vi "Main.vi"() -> ()   [LabVIEW 2019]
doc: "This template is for the Queued Message Handler design pattern.\n\nThe Event Handling Loop generates messages based on user interface actions.\n\nThe Message Handling Loop processes messages generated by the Event Handling Loop, or by other messages. The messages are string values, so new messages can be added easily to the Message Cases case structure in the Message Handling Loop. Each message cluster can also provide an optional value for Message Data, which is a variant that can be converted to whatever message-specific data is required."
uses:
  support/Message Queue/Message Cluster.ctl
  controls/UI Refs.ctl
  Settings/Settings.ctl
  Settings/Runtime Conf.ctl
  controls/UI State.ctl
  Acquisition/HeatFlow/HeatFlow Acq Data.ctl
  <extravilib>/ChannelInstances/Stream-var/Read With Abort.vi
  <extravilib>/ChannelInstances/Messenger-t'Message Queue.lvlib-Message Cluster.ctl'/Write With Abort.vi
  <extravilib>/ChannelInstances/Stream-var/EndpointRead.vi
  <resource>/Channels/Messenger/Write With Abort.vi
  <extravilib>/ChannelInstances/Messenger-t'Message Queue.lvlib-Message Cluster.ctl'/Wrapper.lvclass
  C:/Program Files (x86)/National Instruments/LabVIEW 2019/vi.lib/ChannelSupport/Channel Message/Channel Message.lvclass
  <extravilib>/ChannelInstances/Stream-var/Instantiate.vi
  <extravilib>/ChannelInstances/Stream-var/)Channel.vi
  <resource>/ChannelSupport/_ChannelSupport/WaitIfNeeded.vi
  <extravilib>/ChannelInstances/Messenger-t'Message Queue.lvlib-Message Cluster.ctl'/Instantiate.vi
  <extravilib>/ChannelInstances/Messenger-t'Message Queue.lvlib-Message Cluster.ctl'/Wrap.vi
  <resource>/Channels/Messenger/Endpoint.vi
  <extravilib>/ChannelInstances/Event Messenger-bool/Instantiate.vi
  <extravilib>/ChannelInstances/Event Messenger-bool/))Channel.vi
  <vilib>/Utility/error.llb/Error Cluster From Error Code.vi
  <vilib>/ErrorRing/Error Ring.xnode
  <extravilib>/ChannelInstances/Event Messenger-bool.lvlib
  support/Message Queue/Message Queue.lvlib
  <extravilib>/ChannelInstances/Messenger-t'Message Queue.lvlib-Message Cluster.ctl'.lvlib
  Settings/Settings.lvlib
  Acquisition/Acquisition.lvlib
  Logging/Logging.lvlib
  <extravilib>/ChannelInstances/Stream-var.lvlib
panel:
  out "Jaka wartoœæ":dbl
  in  "ColdSideVolts":dbl min=0.0 max=8.0 step=0.01
  in  "HotSideVolts":dbl min=0.0 max=8.0 step=0.01
  out "Operating Mode":string
  in  "Tab Control":enum32{"Page 1", "Page 2"}(tab)
  out "Heater dU":dbl format="%#.3f"
  out "Hot Side I":dbl format="%#.3f"
  out "I Res dU":dbl format="%#.1f"
  in  "Load Resistance":dbl=3.0 min=0.01 max=100000.0 step=1.0 format="%#.2f"
  out "Load Voltage":dbl format="%#.2f"
  in  "R Check":dbl=5.0 min=0.01 max=100000.0 step=1.0 format="%#.2f"
  in  "s":bool
  out "Boolean":bool
  out "Boolean 2":bool
  in  "s 2":bool
  out "Boolean 3":bool
  out "Boolean 4":bool
  out "Output Power":dbl format="%#.2f"
  out "Output Current":dbl format="%#.0f"
  out "Current above limit":bool
  out "Hot Side Power":dbl format="%9.2f"
  out "Hot Side Temp":dbl format="%#.2f"
  out "Cold Side Temp":dbl format="%#.2f"
  out "T 1":dbl
  out "T 2":dbl
  out "T 3":dbl
  out "T 4":dbl
  out "T 5":dbl
  out "T 6":dbl
  out "T 7":dbl
  out "T 8":dbl
  out "Time Stamp":timestamp
  out "Time Delta ms":u32
  in  "Save Conf File":bool
  out "Config File":string
  in  "Select Config File":bool
  out "Status":string
  out "Current Time Interval, s":dbl
  in  "Update Runtime":bool
  in  "Time Interval, s":dbl=1.0
  in  "Stop Acquisition":bool
  in  "Log all signals":bool
  in  "Start Acquisition":bool
  in  "Exit":bool
  # "K"
  # "K"
  # "W"
  # "mV"
  # "A"
  # "V"
  # "V"
  # "Ohm"
  # "Pomiar Rw"
  # "10 000 Ohm"
  # "W"
  # "Ohm"
  # "mA"
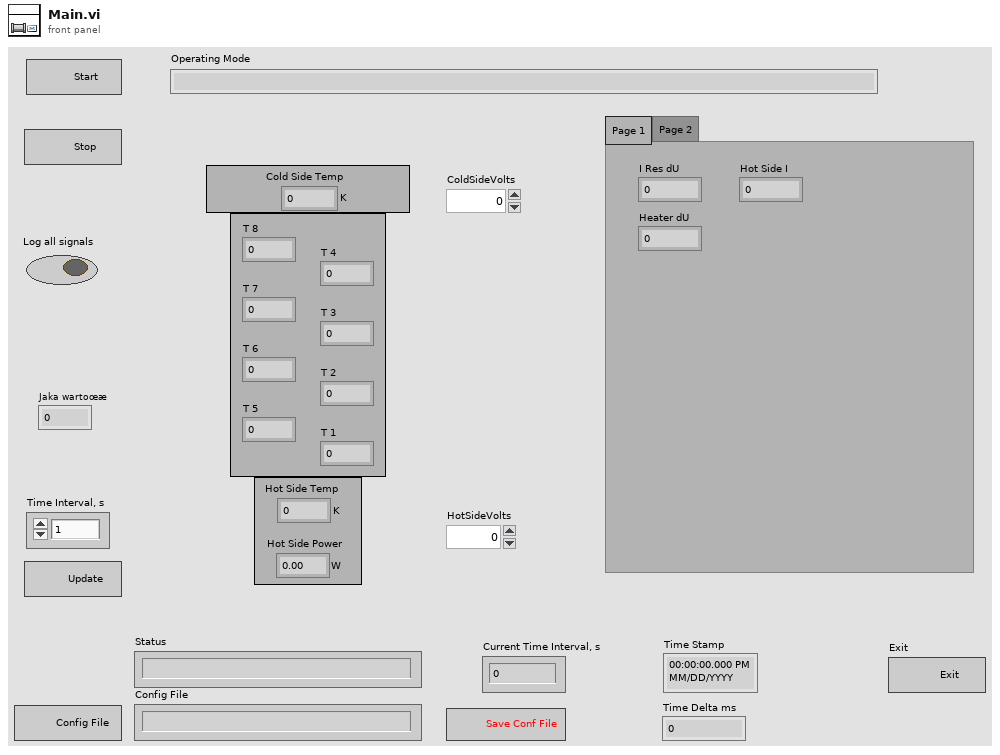
[diagram p1: front panel]
types:
  T1 = typedef "UI State.ctl" = enum16{"Idle", "Acquiring and Logging", "Waiting for Exit", "Waiting for Exit (Acq Stopped)", "Waiting for Exit (Log Stopped)", "Waiting for Stop", "Waiting for Stop (Acq Stopped)", "Waiting for Stop (Log Stopped)"}
  T2 = typedef "Settings.lvlib/Settings.ctl" = cluster{"Runtime":T3, "Cfg Files Dir":path, "Cfg File":path}
  T3 = typedef "Settings.lvlib/Runtime Conf.ctl" = cluster{"Time Interval, s":dbl, "Time Resolution, ms":u32, "Hot Side MOS, V":dbl, "Cold Side MOS, V":dbl}
  T4 = typedef "UI Refs.ctl" = cluster{"Start Acq Ref":refnum<vi>, "Log All Ref":refnum<vi>, "Exit Ref":refnum<vi>, "Stop Acq Ref":refnum<vi>, "Update Ref":refnum<vi>, "Select Config File":refnum<vi>, "Save Config File":refnum<vi>}
  T5 = typedef "Message Queue.lvlib/Message Cluster.ctl" = cluster{"Message":string, "Message Data":variant}
  T6 = typedef "Messenger-t'Message Queue.lvlib-Message Cluster.ctl'.lvlib/))Channel.ctl" = refnum<queue>
  T7 = typedef "Event Messenger-bool.lvlib/))Channel.ctl" = refnum<queue>
  T8 = typedef "Stream-var.lvlib/)Channel.ctl" = refnum<queue>
  T9 = typedef "Acquisition.lvlib/HeatFlow Acq Data.ctl" = cluster{"Time Stamp":timestamp, "Time Delta":u32, "LakeShore_Temp":cluster{"Tube_T_1":dbl, "Tube_T_2":dbl, "Tube_T_3":dbl, "Tube_T_4":dbl, "Tube_T_5":dbl, "Tube_T_6":dbl, "Tube_T_7":dbl, "Tube_T_8":dbl}, "Heaters":cluster{"I_Res_dU":dbl, "Heater_dU":dbl, "Hot_Side_I":dbl, "Hot_Side_P":dbl, "Cold_Ctrl_U":dbl, "Hot_Ctrl_U":dbl, "Hot_Side_T":dbl, "Cold_Side_T":dbl}, "TEG":cluster{"TEG_Load_dU":dbl, "TEG_Load_R":dbl, "TEG_Load_I":dbl, "TEG_Load_P":dbl, "TEG_eta":dbl, "TEG_dT":dbl, "TEG_U_open":dbl, "TEG_U_Test":dbl, "TEG_R_Test":dbl, "TEG_Rw":dbl}, "LastElement?":bool}
  T10 = cluster{"Tube_T_1":dbl, "Tube_T_2":dbl, "Tube_T_3":dbl, "Tube_T_4":dbl, "Tube_T_5":dbl, "Tube_T_6":dbl, "Tube_T_7":dbl, "Tube_T_8":dbl}
  T11 = cluster{"I_Res_dU":dbl, "Heater_dU":dbl, "Hot_Side_I":dbl, "Hot_Side_P":dbl, "Cold_Ctrl_U":dbl, "Hot_Ctrl_U":dbl, "Hot_Side_T":dbl, "Cold_Side_T":dbl}
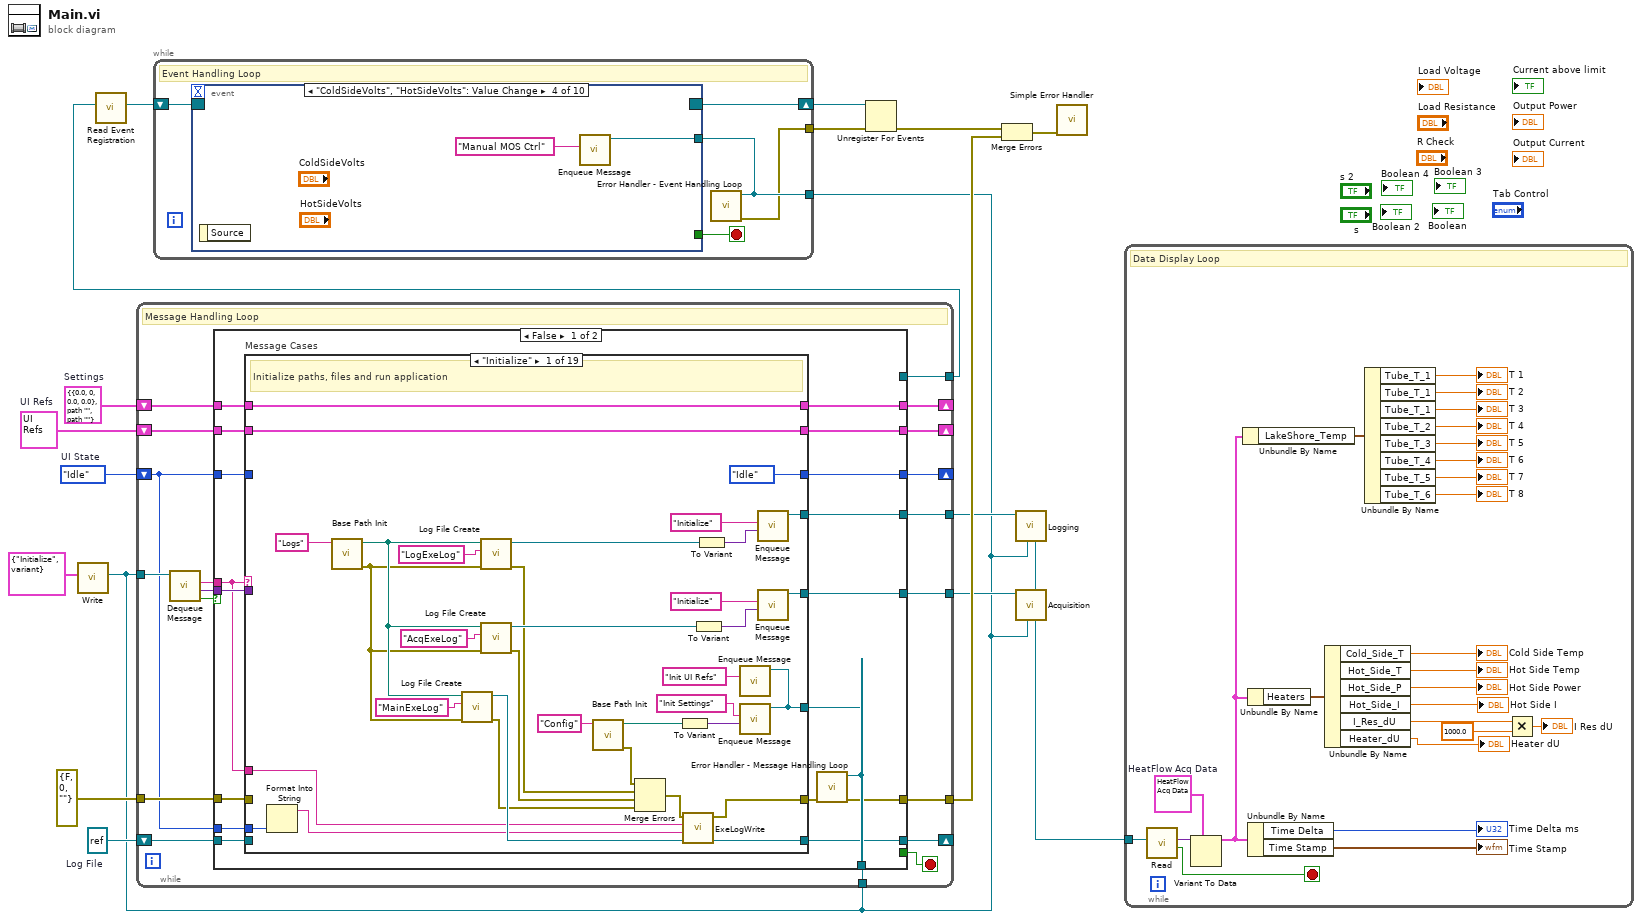
[diagram p0: block diagram]
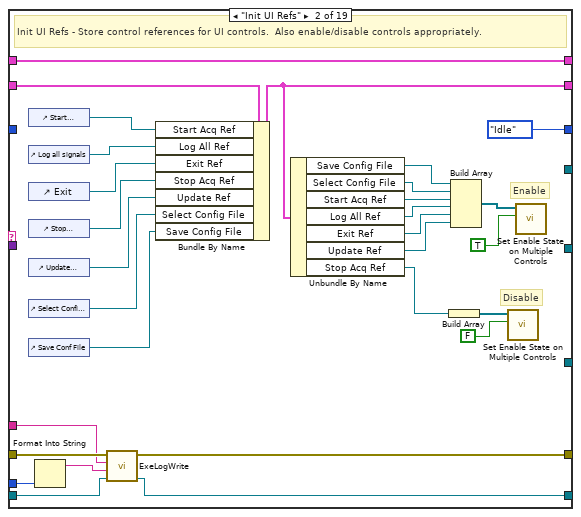
[diagram p2: hidden frame]
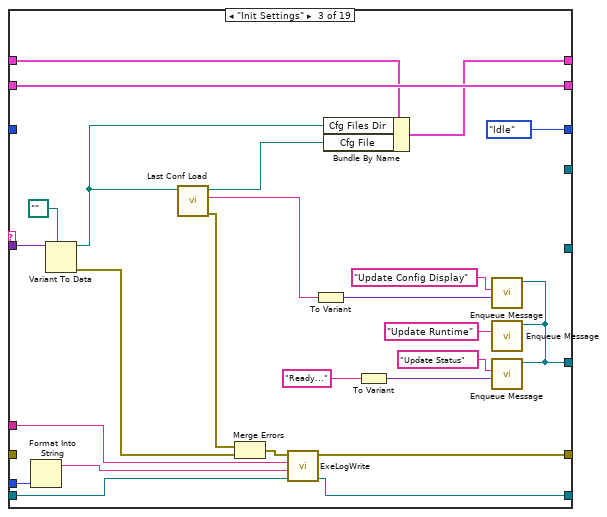
[diagram p3: hidden frame]
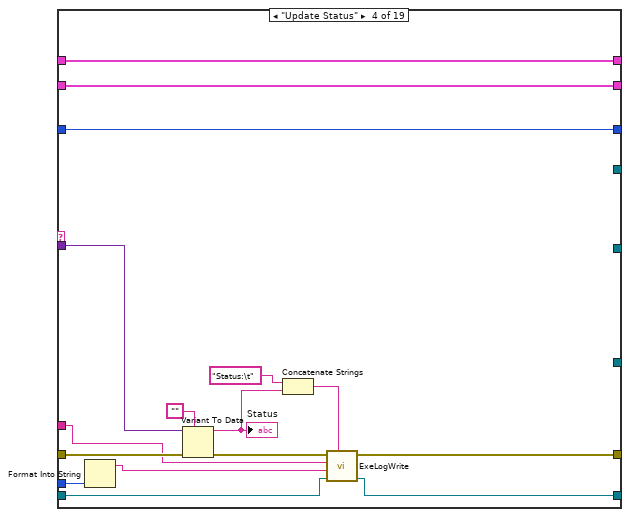
[diagram p4: hidden frame]
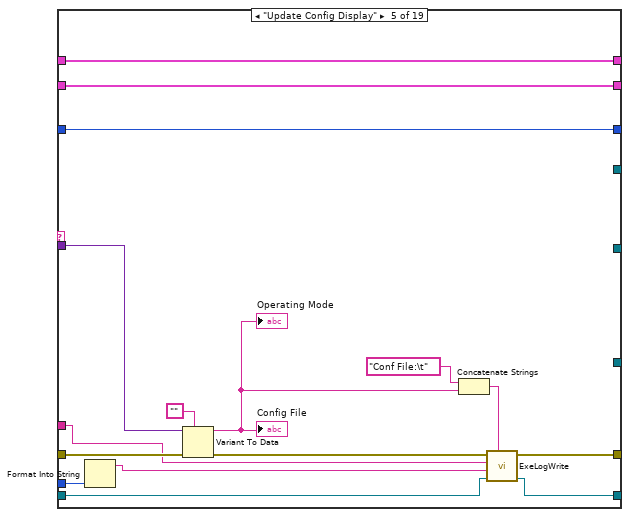
[diagram p5: hidden frame]
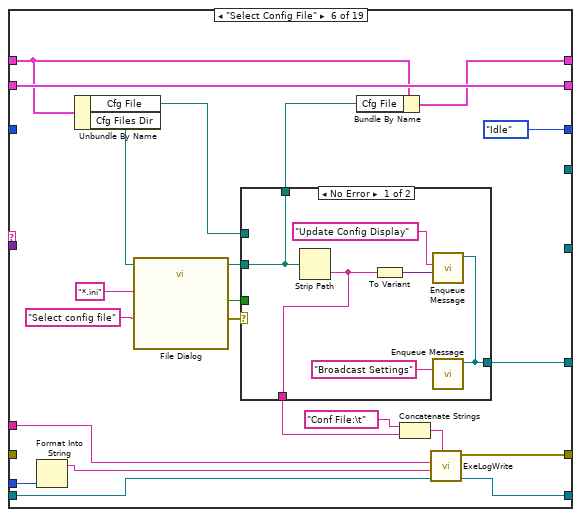
[diagram p6: hidden frame]
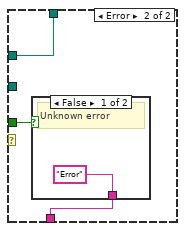
[diagram p7: hidden frame]
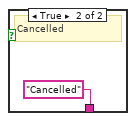
[diagram p8: hidden frame]
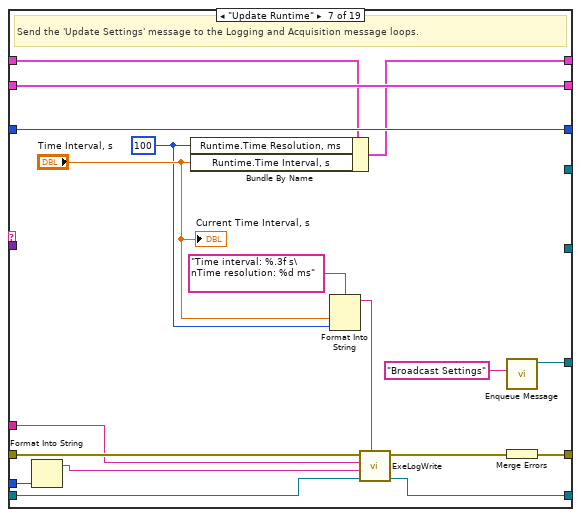
[diagram p9: hidden frame]
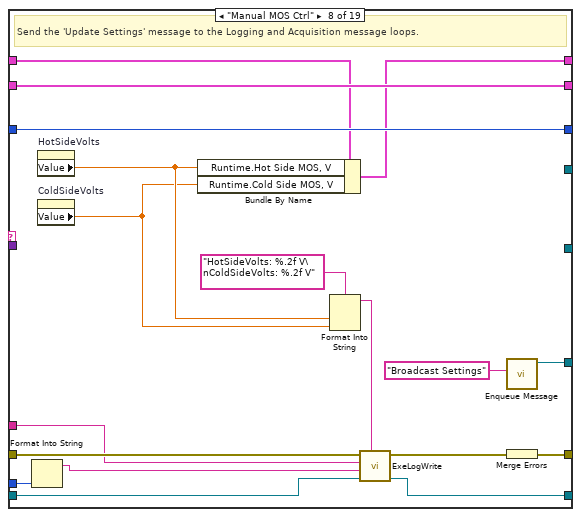
[diagram p10: hidden frame]
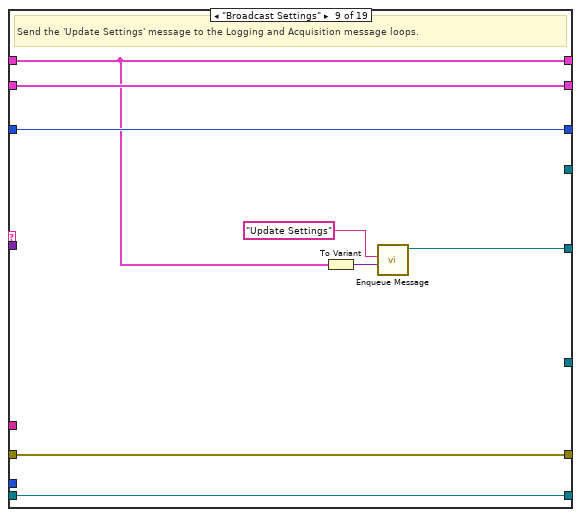
[diagram p11: hidden frame]
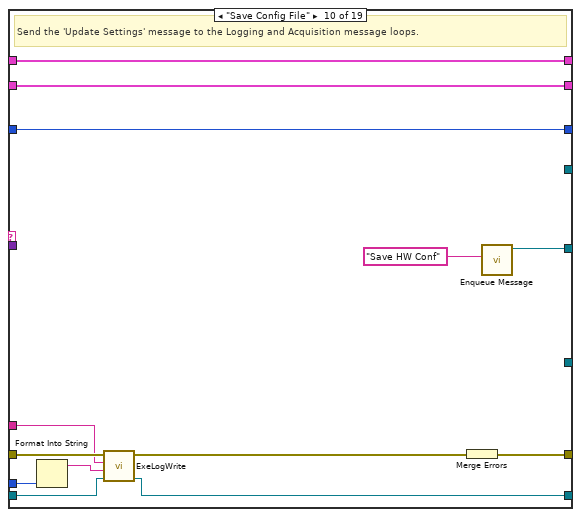
[diagram p12: hidden frame]
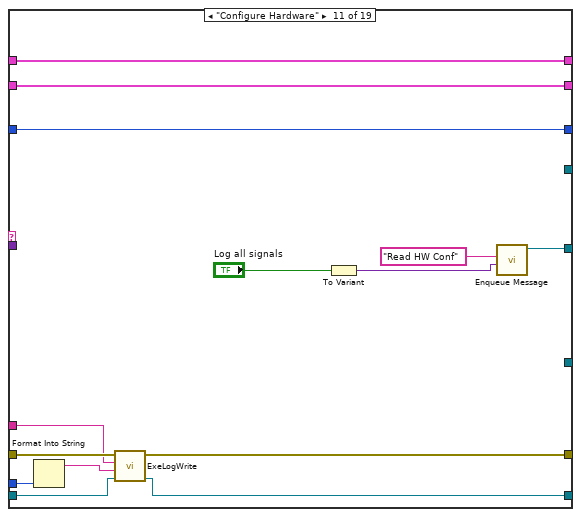
[diagram p13: hidden frame]
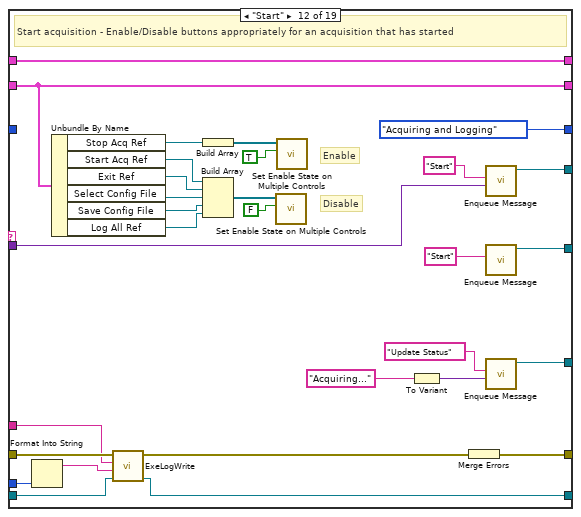
[diagram p14: hidden frame]
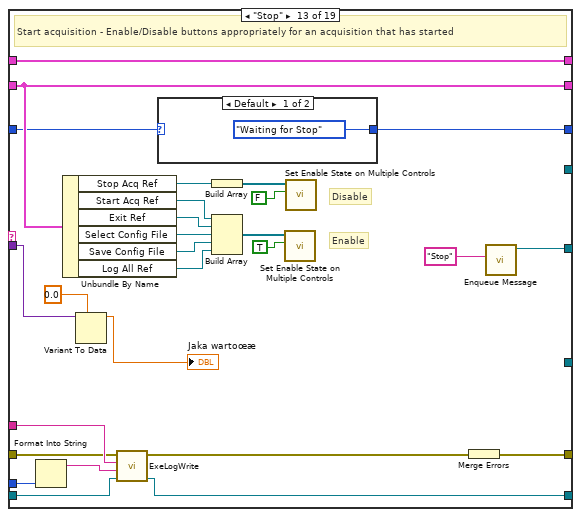
[diagram p15: hidden frame]
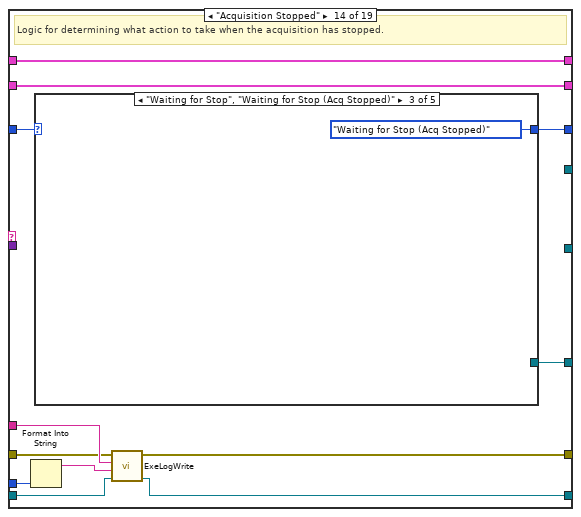
[diagram p17: hidden frame]
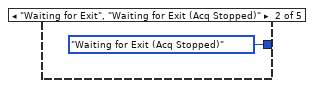
[diagram p19: hidden frame]
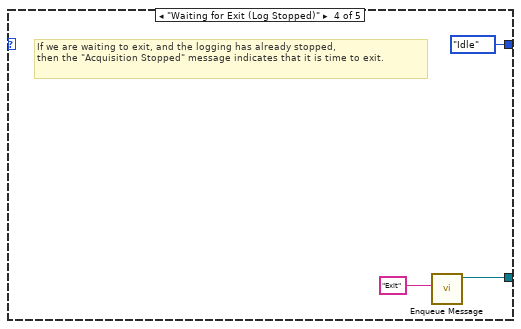
[diagram p20: hidden frame]
diagram:
  w5 = refnum<file> refnum  # Log File
  w10 = UI_State."Idle"  # UI State
  w11 = T2 {"Runtime"={"Time Interval, s"=0.0, "Time Resolution, ms"=0, "Hot Side MOS, V"=0.0, "Cold Side MOS, V"=0.0}, "Cfg Files Dir"=path "", "Cfg File"=path ""}  # Settings
  w12 = T4 {"Start Acq Ref"=refnum, "Log All Ref"=refnum, "Exit Ref"=refnum, "Stop Acq Ref"=refnum, "Update Ref"=refnum, "Select Config File"=refnum, "Save Config File"=refnum}  # UI Refs
  n1 = call <extravilib>:"Write.vi"("element"=T5 {"Message"="Initialize", "Message Data"=variant}) -> ("channel"=w3:T6)  [unwired: 8 in, 2 out]
  n2 = while {
    tunnel: [w37] -> w9
    tunnel: [w36] -> w16
    tunnel: w3 -> [w33]
    tunnel: errorcluster {"status"=FALSE, "code"=0, "source"=""} ("error IO") -> [w35]
    tunnel: w3 -> [w34]
    shift-right: [w28] -> _
    shift-left: w12 -> [w29]
    shift-right: [w26] -> _
    shift-left: w11 -> [w27]
    shift-right: [w25] -> _
    shift-left: w10 -> [w21]
    tunnel: [w24] -> w4
    tunnel: [w23] -> w7
    shift-right: [w19] -> _
    shift-left: w5 -> [w20]
    stop <- w22 stop-if-true
    # "Message Handling Loop"
    n3 = call "Dequeue Message.vi"("channel"=w33) -> ("channel aborted"=w30:bool, "message data"=w31:variant, "message"=w32:string)  [unwired: 8 in]
    n4 = case shown="False" w30 {
      tunnel: [_ TRUE] -> w22
      tunnel: [w54 w471] -> w37
      tunnel: [_ w478] -> w36
      tunnel: w32 -> [w41 _]
      tunnel: w31 -> [w52 w480]
      tunnel: w35 -> [w51 w472]
      tunnel: [w50 _] -> w34
      tunnel: w29 -> [w49 w477]
      tunnel: [w48 w477] -> w28
      tunnel: w27 -> [w47 w476]
      tunnel: [w46 w476] -> w26
      tunnel: w21 -> [w45 w475]
      tunnel: [w44 w475] -> w25
      tunnel: [w43 _] -> w24
      tunnel: [w42 _] -> w23
      tunnel: w21 -> [w38 w474]
      tunnel: w20 -> [w40 w470]
      tunnel: [w39 w469] -> w19
      frame False {
        n5 = case "Message Cases" shown="\"Initialize\"" w41 {
          selector: w41 -> [_ _ _ _ _ _ _ _ _ _ _ _ _ _ _ _ _ _ w459]
          tunnel: w51 -> [_ w98 _ w156 w172 _ w218 w236 w245 w258 w275 w289 w319 w341 w363 _ w405 _ _]
          tunnel: [w59 w93 w127 w150 w166 w189 w225 w243 w245 w264 w274 w308 w335 w339 w361 w396 w404 w440 w460] -> w53
          tunnel: w52 -> [_ _ w138 w157 w173 _ _ _ _ _ _ w281 w311 _ _ w398 _ _ _]
          tunnel: [w84 _ w118 _ _ w179 w208 w228 _ _ _ w294 _ w345 w367 w382 w409 w444 _] -> w50
          tunnel: w49 -> [w87 w115 w140 w155 w171 w196 w224 w242 w251 w263 w268 w302 w331 w348 w370 w395 w412 w445 w458]
          tunnel: [w87 w108 w140 w155 w171 w196 w224 w242 w251 w263 w268 w302 w331 w348 w370 w395 w412 w445 w458] -> w48
          tunnel: w47 -> [w58 w117 w125 w154 w170 w186 w221 w239 w246 w252 w269 w306 w333 w349 w371 w394 w413 w435 w457]
          tunnel: [w58 w117 w124 w154 w170 w185 w220 w238 w246 w252 w269 w306 w333 w349 w371 w394 w413 w435 w457] -> w46
          tunnel: w45 -> [_ _ _ w153 w169 _ w223 w241 w250 w262 w267 _ w324 w347 w369 w393 w411 _ w456]
          tunnel: [UI_State."Idle" ("UI State") UI_State."Idle" ("UI State") UI_State."Idle" ("UI State") w153 w169 UI_State."Idle" ("UI State") w223 w241 w250 w262 w267 UI_State."Acquiring and Logging" ("UI State") w323 w346 w368 w393 w410 UI_State."Idle" ("UI State") w456] -> w44
          tunnel: [w82 _ _ _ _ _ _ _ w249 w261 w277 w303 w332 _ _ _ _ w452 _] -> w43
          tunnel: [w83 _ _ _ _ _ _ _ _ _ _ w304 _ _ _ _ _ w453 _] -> w42
          tunnel: w41 -> [w62 w97 w135 w149 w165 w193 w214 w232 _ w257 w273 w287 w320 w342 w364 w390 w406 w441 _]
          tunnel: w40 -> [_ w95 w133 w147 w163 w191 w216 w234 w244 w255 w271 w285 w317 w340 w362 w389 w403 w439 w455]
          tunnel: [w67 w94 w132 w146 w162 w190 w215 w233 w244 w253 w270 w284 w316 w338 w360 w388 w402 w438 w455] -> w39
          tunnel: w38 -> [w64 w99 w137 w152 w168 w194 w219 w237 _ w259 w276 w290 w322 w344 w366 w392 w408 w443 _]
          frame "Initialize" {
            # "Initialize paths, files and run application"
            n6 = Format Into String(w64) -> (resulting string=w63:string)  [unwired: 3 in, 1 out]
            n7 = call "Base Path Init.vi"("Folder name"="Logs" ("name or relative path")) -> ("error out"=w65:errorcluster, "Folder Path"=w69:path)  [unwired: 9 in]
            n8 = call "Log File Create.vi"("error in"=w65, "initial filename"="MainExeLog", "base path"=w69) -> ("error out"=w61:errorcluster, "refnum out"=w66:refnum<file>)  [unwired: 7 in]
            n9 = call "Log File Create.vi"("error in"=w65, "initial filename"="LogExeLog", "base path"=w69) -> ("error out"=w56:errorcluster, "refnum out"=w78:refnum<file>)  [unwired: 7 in]
            n10 = call "Log File Create.vi"("error in"=w65, "initial filename"="AcqExeLog", "base path"=w69) -> ("error out"=w57:errorcluster, "refnum out"=w76:refnum<file>)  [unwired: 7 in]
            n11 = call "Base Path Init.vi"("Folder name"="Config") -> ("error out"=w55:errorcluster, "Folder Path"=w71:path)  [unwired: 9 in]
            n12 = Merge Errors(w55, w56, w57, w61) -> (w60:errorcluster)
            n13 = To Variant(anything=w71) -> (Variant=w70:variant)
            n14 = call "ExeLogWrite.vi"("refnum in"=w66, "State"=w63, "Message"=w62, "error in"=w60) -> ("refnum out"=w67:refnum<file>, "error out"=w59:errorcluster)  [unwired: 6 in]
            n15 = To Variant(anything=w76) -> (Variant=w74:variant)
            n16 = To Variant(anything=w78) -> (Variant=w75:variant)
            n17 = call "Enqueue Message.vi"("data (empty)"=w70, "message"="Init Settings" ("Message")) -> ("channel"=w84:T6)  [unwired: 9 in]
            n18 = call "Enqueue Message.vi"("channel"=w84, "message"="Init UI Refs" ("Message")) -> ()  [unwired: 10 in]
            n19 = call "Enqueue Message.vi"("data (empty)"=w75, "message"="Initialize") -> ("channel"=w83:T6)  [unwired: 9 in]
            n20 = call "Enqueue Message.vi"("data (empty)"=w74, "message"="Initialize") -> ("channel"=w82:T6)  [unwired: 9 in]
          }
          frame "Init UI Refs" {
            # "Enable"
            # "Disable"
            # "Init UI Refs - Store control references for UI controls.  Also enable/disable controls appropriately."
            n21 = control-ref of="Start Acquisition"() -> (w114:refnum<vi>)
            n22 = control-ref of="Log all signals"() -> (w113:refnum<vi>)
            n23 = control-ref of="Exit"() -> (w110:refnum<vi>)
            n24 = control-ref of="Stop Acquisition"() -> (w109:refnum<vi>)
            n25 = control-ref of="Update Runtime"() -> (w92:refnum<vi>)
            n26 = control-ref of="Select Config File"() -> (w91:refnum<vi>)
            n27 = control-ref of="Save Conf File"() -> (w90:refnum<vi>)
            n28 = Format Into String(w99) -> (resulting string=w96:string)  [unwired: 3 in, 1 out]
            n29 = call "ExeLogWrite.vi"("refnum in"=w95, "State"=w96, "Message"=w97, "error in"=w98) -> ("refnum out"=w94:refnum<file>, "error out"=w93:errorcluster)  [unwired: 6 in]
            n30 = Bundle By Name(cluster=w115, "Start Acq Ref"=w114, "Log All Ref"=w113, "Exit Ref"=w110, "Stop Acq Ref"=w109, "Update Ref"=w92, "Select Config File"=w91, "Save Config File"=w90) -> (w108:T4)
            n31 = Unbundle By Name(w108) -> ("Save Config File"=w89:refnum<vi>, "Select Config File"=w100:refnum<vi>, "Start Acq Ref"=w104:refnum<vi>, "Log All Ref"=w103:refnum<vi>, "Exit Ref"=w102:refnum<vi>, "Update Ref"=w101:refnum<vi>, "Stop Acq Ref"=w107:refnum<vi>)
            n32 = Build Array(w107) -> (w106:refnum<vi>[])
            n33 = Build Array(w89, w100, w104, w103, w102, w101) -> (w105:refnum<vi>[])
            n34 = call "Set Enable State on Multiple Controls.vi"("Enable?"=FALSE, "Controls"=w106) -> ()  [unwired: 10 in]
            n35 = call "Set Enable State on Multiple Controls.vi"("Enable?"=TRUE, "Controls"=w105) -> ()  [unwired: 10 in]
          }
          frame "Init Settings" {
            n36 = Format Into String(w137) -> (resulting string=w134:string)  [unwired: 3 in, 1 out]
            n37 = Variant To Data(type=path "" ("Folder Path"), Variant=w138) -> (data=w123:path, error out=w120:errorcluster)  [unwired: 1 in]
            n38 = call "Last Conf Load.vi"("Config Dir"=w123) -> ("error out"=w119:errorcluster, "Conf File Name"=w121:string, "Conf File path"=w122:path)  [unwired: 8 in]
            n39 = Merge Errors(w119, w120) -> (w126:errorcluster)
            n40 = call "ExeLogWrite.vi"("refnum in"=w133, "State"=w134, "Message"=w135, "error in"=w126) -> ("refnum out"=w132:refnum<file>, "error out"=w127:errorcluster)  [unwired: 6 in]
            n41 = To Variant(anything=w121) -> (Variant=w130:variant)
            n42 = Bundle By Name(cluster=w125, "Cfg Files Dir"=w123, "Cfg File"=w122) -> (w124:T2)
            n43 = To Variant(anything="Ready...") -> (Variant=w129:variant)
            n44 = call "Enqueue Message.vi"("data (empty)"=w129, "message"="Update Status" ("Message")) -> ("channel"=w118:T6)  [unwired: 9 in]
            n45 = call "Enqueue Message.vi"("channel"=w118, "data (empty)"=w130, "message"="Update Config Display") -> ()  [unwired: 9 in]
            n46 = call "Enqueue Message.vi"("channel"=w118, "message"="Update Runtime" ("Message")) -> ()  [unwired: 10 in]
          }
          frame "Update Status" {
            n47 = Format Into String(w152) -> (resulting string=w148:string)  [unwired: 3 in, 1 out]
            n48 = Variant To Data(error in=w156, type="", Variant=w157) -> (data=w144:string, error out=w151:errorcluster)
            "Status" <- w144
            n49 = Concatenate Strings("Status:\t" ("string"), w144) -> (w143:string)
            n50 = call "ExeLogWrite.vi"("Extra"=w143, "refnum in"=w147, "State"=w148, "Message"=w149, "error in"=w151) -> ("refnum out"=w146:refnum<file>, "error out"=w150:errorcluster)  [unwired: 5 in]
          }
          frame "Update Config Display" {
            n51 = Format Into String(w168) -> (resulting string=w164:string)  [unwired: 3 in, 1 out]
            n52 = Variant To Data(error in=w172, type="", Variant=w173) -> (data=w159:string, error out=w167:errorcluster)
            "Config File" <- w159
            "Operating Mode" <- w159
            n53 = Concatenate Strings("Conf File:\t" ("string"), w159) -> (w160:string)
            n54 = call "ExeLogWrite.vi"("Extra"=w160, "refnum in"=w163, "State"=w164, "Message"=w165, "error in"=w167) -> ("refnum out"=w162:refnum<file>, "error out"=w166:errorcluster)  [unwired: 5 in]
          }
          frame "Select Config File" {
            n55 = Format Into String(w194) -> (resulting string=w192:string)  [unwired: 3 in, 1 out]
            n56 = Unbundle By Name(w186) -> ("Cfg File"=w181:path, "Cfg Files Dir"=w183:path)
            n57 = call "File Dialog"("start path"=w183, "prompt"="Select config file", "pattern (all files)"="*.ini") -> ("selected path"=w182:path, "cancelled"=w175:bool, "error out"=w184:errorcluster)  [unwired: 9 in, 1 out]
            n58 = case shown="No Error" w184 {
              tunnel: w182 -> [w198 _]
              tunnel: w181 -> [_ w205]
              tunnel: [w198 w205] -> w180
              tunnel: [w199 _] -> w179
              tunnel: [w197 w203] -> w177
              tunnel: w175 -> [_ w204]
              frame No Error {
                n59 = Strip Path(path=w198) -> (name=w197:string)  [unwired: 1 out]
                n60 = To Variant(anything=w197) -> (Variant=w200:variant)
                n61 = call "Enqueue Message.vi"("message"="Broadcast Settings") -> ("channel"=w199:T6)  [unwired: 10 in]
                n62 = call "Enqueue Message.vi"("channel"=w199, "data (empty)"=w200, "message"="Update Config Display") -> ()  [unwired: 9 in]
              }
              frame Error {
                n63 = case shown="False" w204 {
                  tunnel: ["Error" "Cancelled"] -> w203
                  frame False {
                    # "Unknown error"
                  }
                  frame True {
                    # "Cancelled"
                  }
                }
              }
            }
            n64 = Bundle By Name(cluster=w186, "Cfg File"=w180) -> (w185:T2)
            n65 = Concatenate Strings("Conf File:\t" ("string"), w177) -> (w176:string)
            n66 = call "ExeLogWrite.vi"("Extra"=w176, "refnum in"=w191, "State"=w192, "Message"=w193) -> ("refnum out"=w190:refnum<file>, "error out"=w189:errorcluster)  [unwired: 6 in]
          }
          frame "Update Runtime" {
            w211 = u32 100 ("Runtime Configuration.Time Resolution, ms")
            # "Send the 'Update Settings' message to the Logging and Acquisition message loops."
            n67 = Format Into String(w219) -> (resulting string=w213:string)  [unwired: 3 in, 1 out]
            n68 = Bundle By Name(cluster=w221, "Runtime.Time Resolution, ms"=w211, "Runtime.Time Interval, s"="Time Interval, s") -> (w220:T2)
            n69 = Format Into String(format string="Time interval: %.3f s\nTime resolution: %d ms", "Time Interval, s", w211) -> (resulting string=w209:string)  [unwired: 2 in, 1 out]
            n70 = call "ExeLogWrite.vi"("Extra"=w209, "refnum in"=w216, "State"=w213, "Message"=w214, "error in"=w218) -> ("refnum out"=w215:refnum<file>, "error out"=w217:errorcluster)  [unwired: 5 in]
            n71 = call "Enqueue Message.vi"("message"="Broadcast Settings") -> ("channel"=w208:T6)  [unwired: 10 in]
            n72 = Merge Errors(w217) -> (w225:errorcluster)
            "Current Time Interval, s" <- "Time Interval, s"
          }
          frame "Manual MOS Ctrl" {
            # "Send the 'Update Settings' message to the Logging and Acquisition message loops."
            n73 = Format Into String(w237) -> (resulting string=w231:string)  [unwired: 3 in, 1 out]
            n74 = property on="HotSideVolts" class="DigNum (strict)"() -> ("Value"=w227:dbl)  [unwired: 2 in, 2 out]
            n75 = property on="ColdSideVolts" class="DigNum (strict)"() -> ("Value"=w226:dbl)  [unwired: 2 in, 2 out]
            n76 = Bundle By Name(cluster=w239, "Runtime.Hot Side MOS, V"=w227, "Runtime.Cold Side MOS, V"=w226) -> (w238:T2)
            n77 = Format Into String(format string="HotSideVolts: %.2f V\nColdSideVolts: %.2f V", w227, w226) -> (resulting string=w229:string)  [unwired: 2 in, 1 out]
            n78 = call "ExeLogWrite.vi"("Extra"=w229, "refnum in"=w234, "State"=w231, "Message"=w232, "error in"=w236) -> ("refnum out"=w233:refnum<file>, "error out"=w235:errorcluster)  [unwired: 5 in]
            n79 = call "Enqueue Message.vi"("message"="Broadcast Settings") -> ("channel"=w228:T6)  [unwired: 10 in]
            n80 = Merge Errors(w235) -> (w243:errorcluster)
          }
          frame "Broadcast Settings" {
            # "Send the 'Update Settings' message to the Logging and Acquisition message loops."
            n81 = To Variant(anything=w246) -> (Variant=w247:variant)
            n82 = call "Enqueue Message.vi"("data (empty)"=w247, "message"="Update Settings") -> ("channel"=w249:T6)  [unwired: 9 in]
          }
          frame "Save Config File" {
            # "Send the 'Update Settings' message to the Logging and Acquisition message loops."
            n83 = Format Into String(w259) -> (resulting string=w256:string)  [unwired: 3 in, 1 out]
            n84 = call "ExeLogWrite.vi"("refnum in"=w255, "State"=w256, "Message"=w257, "error in"=w258) -> ("refnum out"=w253:refnum<file>, "error out"=w254:errorcluster)  [unwired: 6 in]
            n85 = Merge Errors(w254) -> (w264:errorcluster)
            n86 = call "Enqueue Message.vi"("message"="Save HW Conf") -> ("channel"=w261:T6)  [unwired: 10 in]
          }
          frame "Configure Hardware" {
            n87 = Format Into String(w276) -> (resulting string=w272:string)  [unwired: 3 in, 1 out]
            n88 = call "ExeLogWrite.vi"("refnum in"=w271, "State"=w272, "Message"=w273, "error in"=w275) -> ("refnum out"=w270:refnum<file>, "error out"=w274:errorcluster)  [unwired: 6 in]
            n89 = To Variant(anything="Log all signals") -> (Variant=w265:variant)
            n90 = call "Enqueue Message.vi"("data (empty)"=w265, "message"="Read HW Conf" ("Message")) -> ("channel"=w277:T6)  [unwired: 9 in]
          }
          frame "Start" {
            # "Disable"
            # "Enable"
            # "Start acquisition - Enable/Disable buttons appropriately for an acquisition that has started"
            n91 = Format Into String(w290) -> (resulting string=w286:string)  [unwired: 3 in, 1 out]
            n92 = Unbundle By Name(w302) -> ("Stop Acq Ref"=w301:refnum<vi>, "Start Acq Ref"=w298:refnum<vi>, "Exit Ref"=w283:refnum<vi>, "Select Config File"=w282:refnum<vi>, "Save Config File"=w280:refnum<vi>, "Log All Ref"=w279:refnum<vi>)
            n93 = call "ExeLogWrite.vi"("refnum in"=w285, "State"=w286, "Message"=w287, "error in"=w289) -> ("refnum out"=w284:refnum<file>, "error out"=w288:errorcluster)  [unwired: 6 in]
            n94 = Build Array(w301) -> (w300:refnum<vi>[])
            n95 = Build Array(w298, w283, w282, w280, w279) -> (w297:refnum<vi>[])
            n96 = call "Set Enable State on Multiple Controls.vi"("Enable?"=FALSE, "Controls"=w297) -> ()  [unwired: 10 in]
            n97 = call "Set Enable State on Multiple Controls.vi"("Enable?"=TRUE, "Controls"=w300) -> ()  [unwired: 10 in]
            n98 = To Variant(anything="Acquiring..." ("message")) -> (Variant=w291:variant)
            n99 = Merge Errors(w288) -> (w308:errorcluster)
            n100 = call "Enqueue Message.vi"("data (empty)"=w281, "message"="Start" ("Message")) -> ("channel"=w304:T6)  [unwired: 9 in]
            n101 = call "Enqueue Message.vi"("message"="Start" ("Message")) -> ("channel"=w303:T6)  [unwired: 10 in]
            n102 = call "Enqueue Message.vi"("data (empty)"=w291, "message"="Update Status") -> ("channel"=w294:T6)  [unwired: 9 in]
          }
          frame "Stop" {
            # "Enable"
            # "Disable"
            # "Start acquisition - Enable/Disable buttons appropriately for an acquisition that has started"
            n103 = Format Into String(w322) -> (resulting string=w321:string)  [unwired: 3 in, 1 out]
            n104 = Unbundle By Name(w331) -> ("Stop Acq Ref"=w330:refnum<vi>, "Start Acq Ref"=w327:refnum<vi>, "Exit Ref"=w315:refnum<vi>, "Select Config File"=w314:refnum<vi>, "Save Config File"=w313:refnum<vi>, "Log All Ref"=w312:refnum<vi>)
            n105 = Variant To Data(type=0.0, Variant=w311) -> (data=→"Jaka wartoœæ":dbl)  [unwired: 1 in, 1 out]
            n106 = call "ExeLogWrite.vi"("refnum in"=w317, "State"=w321, "Message"=w320, "error in"=w319) -> ("refnum out"=w316:refnum<file>, "error out"=w318:errorcluster)  [unwired: 6 in]
            n107 = case shown="Default" w324 {
              selector: w324 -> [_ w337]
              tunnel: [UI_State."Waiting for Stop" ("UI State") w337] -> w323
              frame Default {
              }
              frame "Waiting for Exit" {
              }
            }
            n108 = Build Array(w330) -> (w329:refnum<vi>[])
            n109 = Build Array(w327, w315, w314, w313, w312) -> (w326:refnum<vi>[])
            n110 = call "Set Enable State on Multiple Controls.vi"("Enable?"=TRUE, "Controls"=w326) -> ()  [unwired: 10 in]
            n111 = call "Set Enable State on Multiple Controls.vi"("Enable?"=FALSE, "Controls"=w329) -> ()  [unwired: 10 in]
            n112 = Merge Errors(w318) -> (w335:errorcluster)
            n113 = call "Enqueue Message.vi"("message"="Stop" ("Message")) -> ("channel"=w332:T6)  [unwired: 10 in]
          }
          frame "Acquisition Stopped" {
            # "Logic for determining what action to take when the acquisition has stopped."
            n114 = Format Into String(w344) -> (resulting string=w343:string)  [unwired: 3 in, 1 out]
            n115 = case shown="\"Waiting for Stop\", \"Waiting for Stop (Acq Stopped)\"" w347 {
              selector: w347 -> [w350 _ _ _ _]
              tunnel: [w350 UI_State."Waiting for Exit (Acq Stopped)" ("UI State") UI_State."Waiting for Stop (Acq Stopped)" ("UI State") UI_State."Idle" ("UI State") UI_State."Idle" ("UI State")] -> w346
              tunnel: [_ _ _ w354 w356] -> w345
              frame Default {
              }
              frame "Waiting for Exit", "Waiting for Exit (Acq Stopped)" {
              }
              frame "Waiting for Stop", "Waiting for Stop (Acq Stopped)" {
              }
              frame "Waiting for Exit (Log Stopped)" {
                # "If we are waiting to exit, and the logging has already stopped, \nthen the \"Acquisition Stopped\" message indicates that it is time to exit."
                n116 = call "Enqueue Message.vi"("message"="Exit") -> ("channel"=w354:T6)  [unwired: 10 in]
              }
              frame "Waiting for Stop (Log Stopped)" {
                # "If we are waiting to stop, and the logging has already stopped, \nthen the \"Acquisition Stopped\" message indicates that it is time to stop."
                n117 = call "Enqueue Message.vi"("data (empty)"="Ready...", "message"="Update Status" ("Message")) -> ("channel"=w356:T6)  [unwired: 9 in]
              }
            }
            n118 = call "ExeLogWrite.vi"("refnum in"=w340, "State"=w343, "Message"=w342, "error in"=w341) -> ("refnum out"=w338:refnum<file>, "error out"=w339:errorcluster)  [unwired: 6 in]
          }
          frame "Logging Stopped" {
            # "Logic for determining what action to take when the logging has stopped."
            n119 = Format Into String(w366) -> (resulting string=w365:string)  [unwired: 3 in, 1 out]
            n120 = case shown="\"Waiting for Stop (Acq Stopped)\"" w369 {
              selector: w369 -> [w372 _ _ _ _]
              tunnel: [w372 UI_State."Waiting for Exit (Log Stopped)" ("UI State") UI_State."Waiting for Stop (Log Stopped)" ("UI State") UI_State."Idle" ("UI State") UI_State."Idle" ("UI State")] -> w368
              tunnel: [_ _ _ w376 w378] -> w367
              frame Default {
              }
              frame "Waiting for Exit", "Waiting for Exit (Log Stopped)" {
              }
              frame "Waiting for Stop", "Waiting for Stop (Log Stopped)" {
              }
              frame "Waiting for Exit (Acq Stopped)" {
                # "If we are waiting to exit, and the acquisition has already stopped, \nthen the \"Logging Stopped\" message indicates that it is time to exit."
                n121 = call "Enqueue Message.vi"("message"="Exit") -> ("channel"=w376:T6)  [unwired: 10 in]
              }
              frame "Waiting for Stop (Acq Stopped)" {
                # "If we are waiting to stop, and the acquisition has already stopped, \nthen the \"Logging Stopped\" message indicates that it is time to stop."
                n122 = call "Enqueue Message.vi"("data (empty)"="Ready...", "message"="Update Status" ("Message")) -> ("channel"=w378:T6)  [unwired: 9 in]
              }
            }
            n123 = call "ExeLogWrite.vi"("refnum in"=w362, "State"=w365, "Message"=w364, "error in"=w363) -> ("refnum out"=w360:refnum<file>, "error out"=w361:errorcluster)  [unwired: 6 in]
          }
          frame "Error" {
            # "Error - Display an error dialog. This message is sent by the \"Error Handler\" VIs at the end of other loops in this application."
            n124 = Format Into String(w392) -> (resulting string=w391:string)  [unwired: 3 in, 1 out]
            n125 = Variant To Data(type=errorcluster {"status"=FALSE, "code"=0, "source"=""} ("error constant"), Variant=w398) -> (data=w387:errorcluster)  [unwired: 1 in, 1 out]
            n126 = call <vilib>:"Simple Error Handler.vi"("error in (no error)"=w387) -> ()  [unwired: 4 in, 5 out]
            n127 = call "ExeLogWrite.vi"("refnum in"=w389, "State"=w391, "Message"=w390, "error in"=w387) -> ("refnum out"=w388:refnum<file>, "error out"=w386:errorcluster)  [unwired: 6 in]
            n128 = call <vilib>:"Clear Errors.vi"("error in (no error)"=w386) -> ("error out"=w385:errorcluster)  [unwired: 5 in, 1 out]
            n129 = call "Enqueue Message.vi"("data (empty)"="An error occurred. Acquisition stopped.", "message"="Update Status" ("Message")) -> ("channel"=w382:T6)  [unwired: 9 in]
            n130 = case shown="\"Acquiring and Logging\"" w393 {
              tunnel: w382 -> [_ w399]
              frame "Idle", Default {
              }
              frame "Acquiring and Logging" {
                n131 = call "Enqueue Message.vi"("message"="Stop") -> ("channel"=w399:T6)  [unwired: 10 in]
              }
            }
            n132 = Merge Errors(w385) -> (w396:errorcluster)
          }
          frame "Confirm Quit" {
            # "Confirm Quit - Message that can confirm whether or not the user wants to exit the application."
            n133 = case shown="\"Acquiring and Logging\"" w411 {
              tunnel: [UI_State."Idle" ("UI State") w421] -> w410
              tunnel: [w416 w422] -> w409
              tunnel: ["Ack:\tUnnecessary" ("format string") w418] -> w401
              frame Default {
                # "If 'Confirm Quit' comes in while the system is idle, there is no need for a confirmation message."
                n134 = call "Enqueue Message.vi"("message"="Exit") -> ("channel"=w416:T6)  [unwired: 10 in]
              }
              frame "Acquiring and Logging" {
                n135 = Two Button Dialog(message="Are you sure you want to quit\nwhile the acquisition is running?", 1:"No" ("F button name (\"Cancel\")"), 2:"Yes" ("T button name (\"OK\")")) -> (T button?=w419:bool)
                n136 = Format Into String(format string="Ack:\t%s", w419) -> (resulting string=w418:string)  [unwired: 2 in, 1 out]
                n137 = case shown="True" w419 {
                  tunnel: [_ w429] -> w422
                  tunnel: [UI_State."Acquiring and Logging" ("UI State") UI_State."Waiting for Exit" ("UI State")] -> w421
                  frame False {
                    # "User did not want to quit."
                  }
                  frame True {
                    n138 = call "Enqueue Message.vi"("message"="Stop") -> ("channel"=w429:T6)  [unwired: 10 in]
                  }
                }
              }
            }
            n139 = Format Into String(w408) -> (resulting string=w407:string)  [unwired: 3 in, 1 out]
            n140 = call "ExeLogWrite.vi"("Extra"=w401, "refnum in"=w403, "State"=w407, "Message"=w406, "error in"=w405) -> ("refnum out"=w402:refnum<file>, "error out"=w404:errorcluster)  [unwired: 5 in]
          }
          frame "Exit" {
            w451 = "Exit" ("message")
            # "Enable All"
            n141 = Format Into String(w443) -> (resulting string=w442:string)  [unwired: 3 in, 1 out]
            n142 = Unbundle By Name(w445) -> ("Start Acq Ref"=w448:refnum<vi>, "Log All Ref"=w447:refnum<vi>, "Exit Ref"=w446:refnum<vi>, "Update Ref"=w437:refnum<vi>, "Stop Acq Ref"=w436:refnum<vi>, "Select Config File"=w431:refnum<vi>, "Save Config File"=w430:refnum<vi>)
            n143 = Unbundle By Name(w435) -> ("Cfg Files Dir"=w433:path, "Cfg File"=w432:path)
            n144 = call "Last Conf Save.vi"("Conf Dir"=w433, "Conf File"=w432) -> ("error out"=w434:errorcluster)  [unwired: 7 in]
            n145 = Build Array(w448, w447, w446, w437, w436, w431, w430) -> (w449:refnum<vi>[])
            n146 = call "Set Enable State on Multiple Controls.vi"("Enable?"=TRUE, "Controls"=w449) -> ()  [unwired: 10 in]
            n147 = call "ExeLogWrite.vi"("refnum in"=w439, "State"=w442, "Message"=w441, "error in"=w434) -> ("refnum out"=w438:refnum<file>, "error out"=w440:errorcluster)  [unwired: 6 in]
            n148 = call "Abort Message Queue.vi"() -> ("channel"=w444:T6)  [unwired: 11 in]
            n149 = call "Enqueue Message.vi"("message"=w451) -> ("channel"=w453:T6)  [unwired: 10 in]
            n150 = call "Enqueue Message.vi"("message"=w451) -> ("channel"=w452:T6)  [unwired: 10 in]
          }
          frame Default {
            # "'Default' case only runs if there is a message that isn't defined in any of the other cases.  Output a programming error."
            n151 = xnode "Error Ring"("parameter 0"=w459) -> ("error out"=w460:errorcluster)
          }
        }
        n152 = call "Error Handler - Message Handling Loop.vi"("channel"=w50, "error in (no error)"=w53) -> ("dup error in"=w54:errorcluster)  [unwired: 9 in]
      }
      frame True {
        w479 = TRUE  # Exit
        # "Tell the event loop to stop if it has not done so already."
        # "Ignore error out here. If the Exit message was sent without an attached error, that is fine."
        # "#CodeNeeded - Add any required cleanup code here, such as putting hardware into a safe mode. Note that if 'Exit' was called as a result of an error, an error dialog will be displayed. Add any custom error handling for an 'Exit' condition here as well."
        # "Shutdown routine."
        n153 = Format Into String(w474) -> (resulting string=w473:string)  [unwired: 3 in, 1 out]
        n154 = call "ExeLogWrite.vi"("refnum in"=w470, "State"=w473, "Message"="Shutdown", "error in"=w472) -> ("refnum out"=w469:refnum<file>, "error out"=w471:errorcluster)  [unwired: 6 in]
        n155 = Variant To Data(type=errorcluster {"status"=FALSE, "code"=0, "source"=""} ("error constant"), Variant=w480) -> (data=w481:errorcluster)  [unwired: 1 in, 1 out]
        n156 = call <vilib>:"Simple Error Handler.vi"("error in (no error)"=w481) -> ()  [unwired: 4 in, 5 out]
        n157 = call <extravilib>:"Write.vi"("element"=w479) -> ("channel"=w478:T7)  [unwired: 9 in, 1 out]
      }
    }
  }
  n158 = call <extravilib>:"Read Event Registration.vi"("channel"=w16) -> ("event registration refnum"=w15:refnum<event-registration>)  [unwired: 10 in]
  n159 = while {
    shift-right: [w487] -> w17
    shift-left: w15 -> [w488]
    tunnel: w3 -> [w486]
    tunnel: [w485] -> w8
    stop <- w484 stop-if-true
    # "Event Handling Loop"
    n160 = event shown="[3] \"ColdSideVolts\", \"HotSideVolts\": Value Change" {
      selector: w488 -> [_ _ _ _ _ _ _ _ _ _]
      dyn-events: [_ _ _ _ _ _ _ _ _ _] -> w487
      timeout: _ -> [_ _ _ _ _ _ _ _ _ _]
      tunnel: [_ _ _ _ _ _ _ _ _ TRUE ("Discard?")] -> w484
      tunnel: [w490 w492 w494 w496 w497 w499 w502 _ w505 _] -> w486
      event "Start Acquisition": Value Change {
        n161 = event-data() -> ()  [unwired: 1 in, 1 out]
        n162 = call "Enqueue Message.vi"("message"="Configure Hardware" ("Message")) -> ("channel"=w490:T6)  [unwired: 10 in]
      }
      event "Stop Acquisition": Value Change {
        n163 = event-data() -> ()  [unwired: 1 in, 1 out]
        n164 = call "Enqueue Message.vi"("message"="Stop") -> ("channel"=w492:T6)  [unwired: 10 in]
      }
      event "Update Runtime": Value Change {
        n165 = event-data() -> ()  [unwired: 1 in, 1 out]
        n166 = call "Enqueue Message.vi"("message"="Update Runtime") -> ("channel"=w494:T6)  [unwired: 10 in]
      }
      event "ColdSideVolts", "HotSideVolts": Value Change {
        n167 = event-data() -> ()  [unwired: 1 in, 1 out]
        n168 = call "Enqueue Message.vi"("message"="Manual MOS Ctrl") -> ("channel"=w496:T6)  [unwired: 10 in]
      }
      event "Select Config File": Value Change {
        n169 = event-data() -> ()  [unwired: 1 in, 1 out]
        n170 = call "Enqueue Message.vi"("message"="Select Config File") -> ("channel"=w497:T6)  [unwired: 10 in]
      }
      event "Save Conf File": Value Change {
        n171 = event-data() -> ()  [unwired: 1 in, 1 out]
        n172 = call "Enqueue Message.vi"("message"="Save Config File") -> ("channel"=w499:T6)  [unwired: 10 in]
      }
      event Panel Close? {
        # "Ask user to confirm quit, which will send the exit message if the user says yes. Regardless of the user's response, discard the event so the Exit message has a chance to run to clean up the application."
        n173 = event-data() -> ()  [unwired: 1 in, 1 out]
        n174 = event-data("Discard?"=TRUE) -> ()  [unwired: 1 in, 1 out]
        n175 = call "Enqueue Message.vi"("message"="Confirm Quit") -> ("channel"=w502:T6)  [unwired: 10 in]
      }
      event Application Instance Close {
        # "#CodeRecommended - When a project closes, all VIs within that project are aborted and leave memory. However, any code placed in this event frame is guaranteed to run to completion, so add any cleanup code that absolutely must happen here when working in the development environment. Normal shutdown code should go in the \"aborted=true\" frame in the Message Handling Loop."
        n176 = event-data() -> ()  [unwired: 1 in, 1 out]
      }
      event "Exit": Value Change {
        n177 = event-data() -> ()  [unwired: 1 in, 1 out]
        n178 = call "Enqueue Message.vi"("message"="Exit") -> ("channel"=w505:T6)  [unwired: 10 in]
      }
      event User Event {
        # "The Message Handling Loop processed an \"Exit\" message, which fired this event to stop the Event Handling Loop."
        n179 = event-data() -> ()  [unwired: 1 in, 1 out]
      }
    }
    n180 = call "Error Handler - Event Handling Loop.vi"("channel"=w486) -> ("dup error in"=w485:errorcluster)  [unwired: 10 in]
  }
  n181 = Unregister For Events(event registration refnum=w17, error in=w8) -> (error out=w18:errorcluster)
  n182 = Merge Errors(w18, w9) -> (w6:errorcluster)
  n183 = call "Acquisition.vi"("UI Msg"=w3, "Acq Msg"=w4) -> ("Display Stream"=w2:T8, "Log Stream"=w1:T8)  [unwired: 8 in]
  n184 = call "Logging.vi"("Log Stream"=w1, "UI Msg"=w3, "Log Msg"=w7) -> ()  [unwired: 9 in]
  n185 = call <vilib>:"Simple Error Handler.vi"("error in (no error)"=w6) -> ()  [unwired: 4 in, 5 out]
  n186 = while "Data Display Loop" {
    tunnel: w2 -> [w508]
    stop <- w510 stop-if-true
    w507 = T9 {"Time Stamp"=timestamp(0 s since 1904-01-01), "Time Delta"=0, "LakeShore_Temp"={"Tube_T_1"=0.0, "Tube_T_2"=0.0, "Tube_T_3"=0.0, "Tube_T_4"=0.0, "Tube_T_5"=0.0, "Tube_T_6"=0.0, "Tube_T_7"=0.0, "Tube_T_8"=0.0}, "Heaters"={"I_Res_dU"=0.0, "Heater_dU"=0.0, "Hot_Side_I"=0.0, "Hot_Side_P"=0.0, "Cold_Ctrl_U"=0.0, "Hot_Ctrl_U"=0.0, "Hot_Side_T"=0.0, "Cold_Side_T"=0.0}, "TEG"={"TEG_Load_dU"=0.0, "TEG_Load_R"=0.0, "TEG_Load_I"=0.0, "TEG_Load_P"=0.0, "TEG_eta"=0.0, "TEG_dT"=0.0, "TEG_U_open"=0.0, "TEG_U_Test"=0.0, "TEG_R_Test"=0.0, "TEG_Rw"=0.0}, "LastElement?"=FALSE}  # HeatFlow Acq Data
    # "Data Display Loop"
    n187 = call <extravilib>:"Read.vi"("channel"=w508) -> ("last element?"=w510:bool, "element"=w511:variant)  [unwired: 6 in, 3 out]
    n188 = Variant To Data(type=w507, Variant=w511) -> (data=w509:T9)  [unwired: 1 in, 1 out]
    n189 = Unbundle By Name(w509) -> ("LakeShore_Temp"=w525:T10)
    n190 = Unbundle By Name(w509) -> ("Heaters"=w529:T11)
    n191 = Unbundle By Name(w509) -> ("Time Delta"=→"Time Delta ms":u32, "Time Stamp"=→"Time Stamp":timestamp)
    n192 = Unbundle By Name(w529) -> ("Cold_Side_T"=→"Cold Side Temp":dbl, "Hot_Side_T"=→"Hot Side Temp":dbl, "Hot_Side_P"=→"Hot Side Power":dbl, "Hot_Side_I"=→"Hot Side I":dbl, "I_Res_dU"=w514:dbl, "Heater_dU"=→"Heater dU":dbl)
    n193 = Unbundle By Name(w525) -> ("Tube_T_1"=→"T 1":dbl, "Tube_T_1"=→"T 2":dbl, "Tube_T_1"=→"T 3":dbl, "Tube_T_2"=→"T 4":dbl, "Tube_T_3"=→"T 5":dbl, "Tube_T_4"=→"T 6":dbl, "Tube_T_5"=→"T 7":dbl, "Tube_T_6"=→"T 8":dbl)
    n194 = Multiply(x=w514, y=1000.0) -> (x*y=→"I Res dU":dbl)
  }
